vi "写入EXCEL路径.vi"(8 "error in (no error)":errorcluster caption="错误输入（无错误）", 10 "EXCEL路径":path, 11 "抽取参数输入":refnum<class "抽取参数.lvclass">) -> (0 "error out":errorcluster caption="错误输出", 3 "抽取参数输出":refnum<class "抽取参数.lvclass">)   [LabVIEW 2020, in "抽取参数.lvclass"]
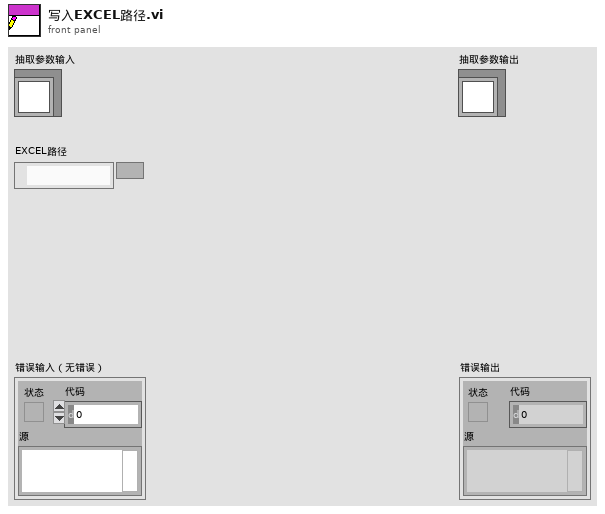
[diagram p1: front panel]
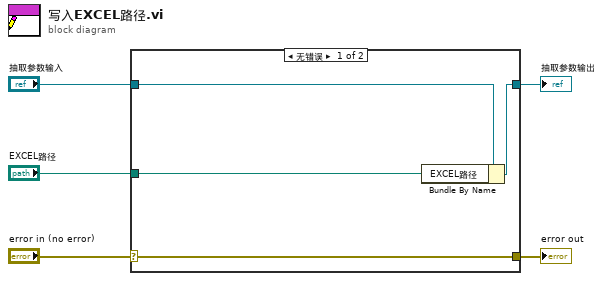
[diagram p0: block diagram]
diagram:
  n1 = case shown="无错误" "error in (no error)" {
    selector: "error in (no error)" -> [w9 w10]
    tunnel: [w9 w10] -> w4
    tunnel: [w7 w11] -> w2
    tunnel: "抽取参数输入" -> [w8 w11]
    tunnel: "EXCEL路径" -> [w6 _]
    frame No Error {
      n2 = Bundle By Name(cluster=w8, "EXCEL路径"=w6) -> (w7:refnum<class "抽取参数.lvclass">)
    }
    frame Error {
    }
  }
  "error out" <- w4
  "抽取参数输出" <- w2
